vi "AccelerometerVoltageSampleLoop.vi"   [LabVIEW 2018]
uses:
  AccelerometerSample.ctl
  <vilib>/rvi/Emulation/niFpgaGetClockAttributes.vi
  <vilib>/rvi/Emulation/niFpgaSctlEmulationGetInTimedLoop.vi
  <vilib>/rvi/Emulation/niFpgaEmulationReportErrorSimple.vi
  <vilib>/rvi/Emulation/niFpgaEmulationIsFPGAContextNoSignature.vi
  <vilib>/rvi/errors/niFpgaSetErrorForExecOnDevCompSimple.vi
  <vilib>/rvi/eio/common/nirviEmuReportErrorAndStop.vi
  <vilib>/rvi/DataTransferAndStorage/Container/Common/niFpgaContainerGetUniqueNameForEmu.vi
  <vilib>/rvi/FIFO/Fifo_Resource/nirvififoEmulationSetSize.vi
  <vilib>/rvi/FIFO/Fifo_Resource/nirviFifoEmulationQueueMgr.vi
  <instcachedir>/0/nirviFifoEmulationQueueMgr_E5CAEC123FF24DC58D834DCA3CDAA9B5.lvgen/nirviFifoEmulationQueueMgr_E5CAEC123FF24DC58D834DCA3CDAA9B5_005.vi
  <vilib>/Utility/error.llb/Clear Errors.vi
  <vilib>/rvi/FIFO/Fifo_Resource/nirvififoEmulationCreateLock.vi
  <vilib>/rvi/Emulation/niFpgaProcessEmulError.vi
  <vilib>/rvi/FIFO/Fifo_Resource/nirvififoEmulationObtainLock.vi
  <vilib>/rvi/FIFO/Fifo_Resource/nirvififoEmulationReleaseLock.vi
  <vilib>/rvi/occurrence/nirviWaitOnOccurrenceBase.vi
  <vilib>/rvi/errors/nirviReportUnexpectedCaseInternalError.vi
  <vilib>/rvi/errors/nirviReportUnexpectedCaseInternalError (U32).vi
  <vilib>/rvi/eio/common/nirviEmuTemplateMethod_errors.vi
  <vilib>/rvi/Memory/Memory_Emulation/niFpgaMemoryEmulationCacheClearOnFirstRun.vi
  <vilib>/rvi/Memory/Memory_Emulation/nirvimemoryEmulationManagerCache_MakeExclusive.vi
  <vilib>/rvi/Memory/Memory_Emulation/niFpgaMemoryEmulationValidateCache.vi
  <vilib>/rvi/Memory/Memory_Emulation/nirvimemoryEmulationManagerCache_InsertValue.vi
  <vilib>/rvi/Memory/Memory_Emulation/nirvimemoryEmulationManagerCache_ReleaseExclusive.vi
  <vilib>/rvi/Memory/Memory_Emulation/nirvimemoryEmulationManagerCache_GetValue.vi
  <vilib>/rvi/Memory/Memory_Emulation/nirvimemoryEmulationManagerCache_SetValue.vi
  <instcachedir>/0/nirviFifoEmulationQueueMgr_E5CAEC123FF24DC58D834DCA3CDAA9B5.lvgen/nirviFifoEmulationQueueMgr_E5CAEC123FF24DC58D834DCA3CDAA9B5_016.vi
  <vilib>/rvi/FIFO/Fifo_Resource/nirvififoEmulationDetermineInputValidOut.vi
  <vilib>/rvi/Emulation/niFpgaCriticalErrorInLSC.vi
  <vilib>/rvi/DataTransferAndStorage/Container/XNode/niFpgaContainer.xnode
  <vilib>/rvi/FIFO/Fifo_Resource/nirvififoEmulationRead.vi
  <vilib>/eio/EIONode/EIONode.xnode
  <vilib>/rvi/DataTransferAndStorage/Register/Emulation/niFpgaRegisterEmulation.vi
  <vilib>/rvi/FIFO/Fifo_Resource/nirvififoEmulationWrite.vi
types:
  T1 = typedef "AccelerometerSample.ctl" = cluster{"Sample":u64, "Timestamp":u64, "Raw1":sgl, "Raw2":sgl, "Raw3":sgl, "Raw4":sgl, "Raw5":sgl, "Raw6":sgl, "Raw7":sgl, "Raw8":sgl}
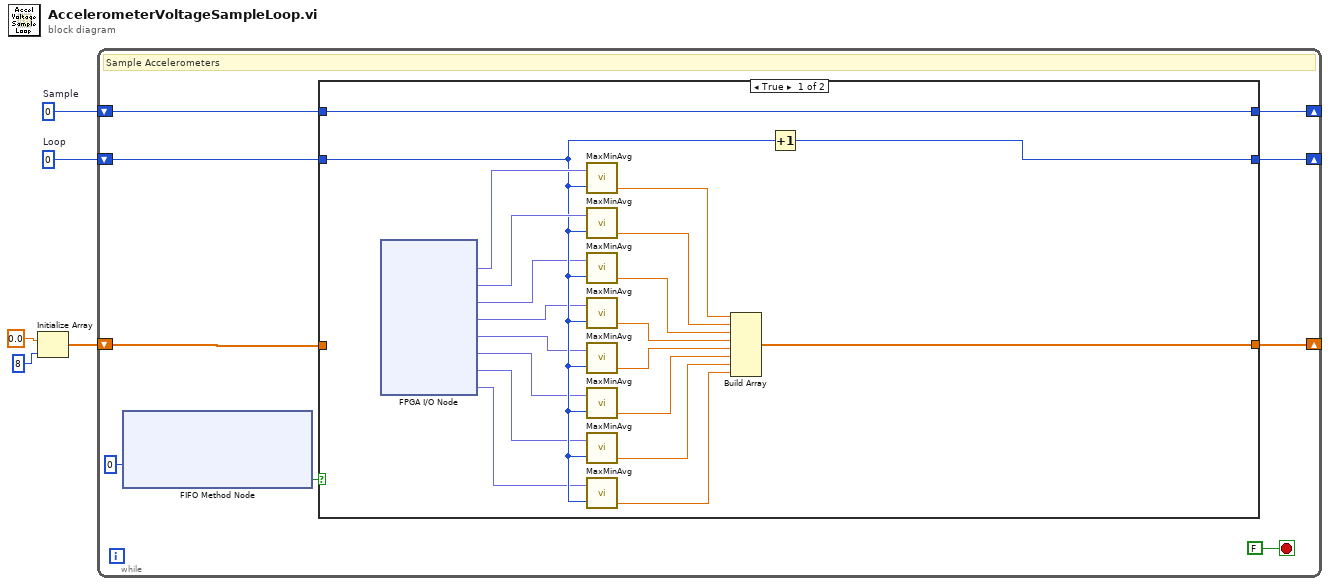
[diagram p0: block diagram]
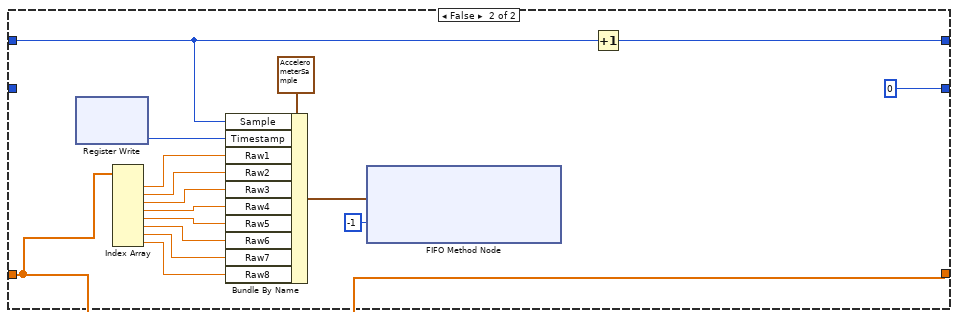
[diagram p2: hidden frame]
diagram:
  w4 = u64 0  # Sample
  w5 = u64 0  # Loop
  n1 = Initialize Array(sgl 0.0 ("element"), 8 ("dimension size")) -> (w1:sgl[])
  n2 = while {
    shift-right: [w10] -> _
    shift-left: w5 -> [w11]
    shift-right: [w8] -> _
    shift-left: w4 -> [w9]
    shift-right: [w6] -> _
    shift-left: w1 -> [w7]
    stop <- FALSE stop-if-true
    # "Sample Accelerometers"
    n3 = xnode ("FIFO Method Node")("Timeout"=0) -> ("Timed Out?"=w13:bool)  [unwired: 1 in, 2 out]
    n4 = case shown="True" w13 {
      tunnel: w11 -> [w28 _]
      tunnel: [w33 u64 0 ("Sample")] -> w10
      tunnel: [w32 w45] -> w8
      tunnel: w9 -> [w32 w44]
      tunnel: [w30 w35] -> w6
      tunnel: w7 -> [_ w35]
      frame True {
        n5 = xnode "FPGA I/O Node"() -> ("Mod1/AI0"=w34:fxp<+/-,24,5>, "Mod1/AI1"=w29:fxp<+/-,24,5>, "Mod1/AI2"=w27:fxp<+/-,24,5>, "Mod1/AI3"=w26:fxp<+/-,24,5>, "Mod2/AI0"=w25:fxp<+/-,24,5>, "Mod2/AI1"=w24:fxp<+/-,24,5>, "Mod2/AI2"=w23:fxp<+/-,24,5>, "Mod2/AI3"=w22:fxp<+/-,24,5>)  [unwired: 8 in, 8 out]
        n6 = call "MaxMinAvg.vi"("Measurement"=w34, "Index"=w28) -> ("Average Value"=w31:sgl)  [unwired: 2 out]
        n7 = call "MaxMinAvg.vi"("Measurement"=w29, "Index"=w28) -> ("Average Value"=w21:sgl)  [unwired: 2 out]
        n8 = call "MaxMinAvg.vi"("Measurement"=w27, "Index"=w28) -> ("Average Value"=w20:sgl)  [unwired: 2 out]
        n9 = call "MaxMinAvg.vi"("Measurement"=w26, "Index"=w28) -> ("Average Value"=w15:sgl)  [unwired: 2 out]
        n10 = call "MaxMinAvg.vi"("Measurement"=w25, "Index"=w28) -> ("Average Value"=w19:sgl)  [unwired: 2 out]
        n11 = call "MaxMinAvg.vi"("Measurement"=w24, "Index"=w28) -> ("Average Value"=w18:sgl)  [unwired: 2 out]
        n12 = call "MaxMinAvg.vi"("Measurement"=w23, "Index"=w28) -> ("Average Value"=w17:sgl)  [unwired: 2 out]
        n13 = call "MaxMinAvg.vi"("Measurement"=w22, "Index"=w28) -> ("Average Value"=w16:sgl)  [unwired: 2 out]
        n14 = Build Array(w31, w21, w20, w15, w19, w18, w17, w16) -> (w30:sgl[])
        n15 = Increment(x=w28) -> (x+1=w33:u64)
      }
      frame False {
        n16 = xnode "Register Write"() -> ("Data"=w47:u64)  [unwired: 1 in, 1 out]
        n17 = Index Array(array=w35) -> (element #1=w43:sgl, element #2=w42:sgl, element #3=w41:sgl, element #4=w40:sgl, element #5=w39:sgl, element #6=w38:sgl, element #7=w37:sgl, element #8=w36:sgl)  [unwired: 8 in]
        n18 = Bundle By Name(cluster=T1 {"Sample"=0, "Timestamp"=0, "Raw1"=0.0, "Raw2"=0.0, "Raw3"=0.0, "Raw4"=0.0, "Raw5"=0.0, "Raw6"=0.0, "Raw7"=0.0, "Raw8"=0.0} ("AccelerometerSample"), "Sample"=w44, "Timestamp"=w47, "Raw1"=w43, "Raw2"=w42, "Raw3"=w41, "Raw4"=w40, "Raw5"=w39, "Raw6"=w38, "Raw7"=w37, "Raw8"=w36) -> (w50:T1)
        n19 = xnode ("FIFO Method Node")("Element"=w50, "Timeout"=-1) -> ()  [unwired: 1 in, 2 out]
        n20 = Increment(x=w44) -> (x+1=w45:u64)
      }
    }
  }
